vi "getDate.vi"(8 "error in (no error)":errorcluster, 11 "Shift in":refnum<class "Shift.lvclass">) -> (0 "error out":errorcluster, 2 "Date":string, 3 "Shift out":refnum<class "Shift.lvclass">)   [LabVIEW 2013, in "Shift.lvclass"]
uses:
  Shift.lvclass
  Shift.lvclass/Shift.ctl
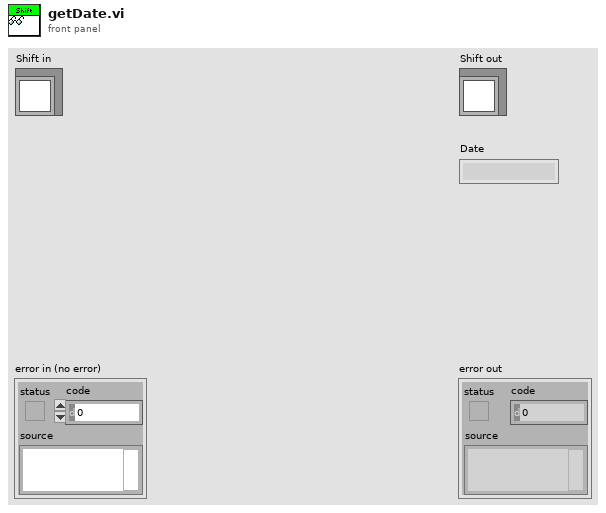
[diagram p1: front panel]
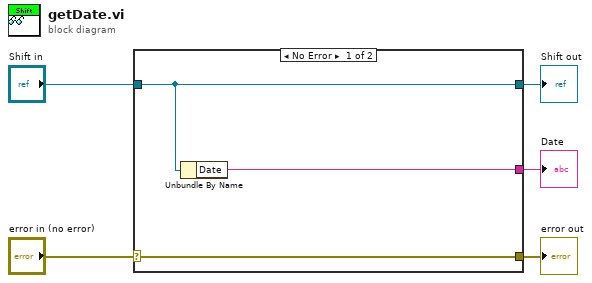
[diagram p0: block diagram]
diagram:
  n1 = case shown="No Error" "error in (no error)" {
    selector: "error in (no error)" -> [w8 w9]
    tunnel: [w8 w9] -> w4
    tunnel: [w7 w10] -> w2
    tunnel: "Shift in" -> [w7 w10]
    tunnel: [w6 _] -> w1
    frame No Error {
      n2 = Unbundle By Name(w7) -> ("Date"=w6:string)
    }
    frame Error {
    }
  }
  "error out" <- w4
  "Shift out" <- w2
  "Date" <- w1
